vi "Wait.Gui.UpdateMsg.vi"(8 "error in (no error)":errorcluster, 10 "Status":string) -> (0 "error out":errorcluster)   [LabVIEW 2016]
uses:
  Wait.Gui.Action.ctl
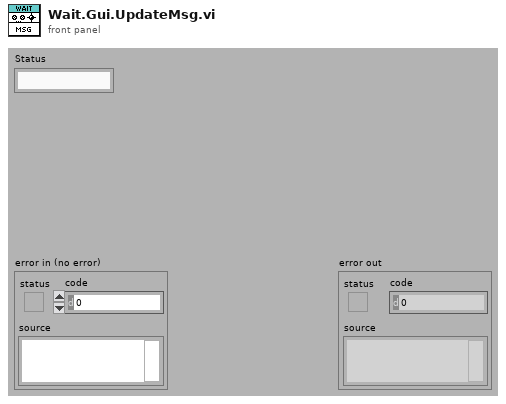
[diagram p1: front panel]
types:
  T1 = typedef "Wait.Gui.Action.ctl" = enum32{"idle", "constructor", "destructor", "--- GuiServerWait ---", "open FP", "close FP", "update msg", "update progbar"}
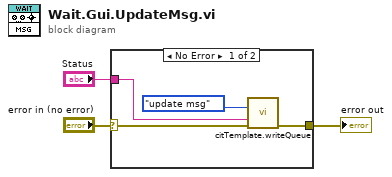
[diagram p0: block diagram]
diagram:
  n1 = case shown="No Error" "error in (no error)" {
    selector: "error in (no error)" -> [w4 w8]
    tunnel: "Status" -> [w6 _]
    tunnel: [w5 w8] -> w2
    frame No Error {
      n2 = call "citTemplate.writeQueue.vi"("event in (if not connected:all statemachine with data event)"=Wait.Gui.Action."update msg" ("Action"), "data in"=w6, "error in (no error)"=w4) -> ("error out"=w5:errorcluster)  [unwired: 12 in]
    }
    frame Error {
    }
  }
  "error out" <- w2
